vi "Set Editor Mode.vi"(8 "Error In":errorcluster, 10 "Mode in":T1, 11 "object in":refnum<class "WebView.JSONEditor.lvclass">) -> (0 "Error Out":errorcluster, 3 "object out":refnum<class "WebView.JSONEditor.lvclass">)   [LabVIEW 2020, in "WebView.JSONEditor.lvclass"]
uses:
  WebView.JSONEditor.lvclass
  <vilib>/JDP Science/JSONtext/LVClass Serializer/JSONtext LVClass Serializer.lvclass
  WebView_class/WebView.lvclass
  f8653de4-75b8-4eba-bbea-61abc822b106.vi
  WebView_class/Editor Mode--enum.ctl
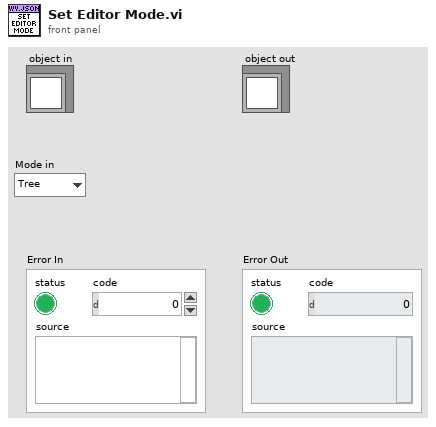
[diagram p1: front panel]
types:
  T1 = typedef "WebView.JSONEditor.lvclass/Editor Mode--enum.ctl" = enum16{"Tree", "View", "Form", "Code", "Text"}
  T2 = cluster{"type":enum16{"loadJSON", "setMode", "getJSON"}, "mode":string}
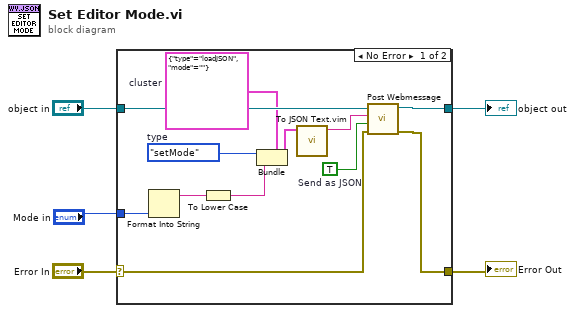
[diagram p0: block diagram]
diagram:
  n1 = case shown="No Error" "Error In" {
    selector: "Error In" -> [w8 w19]
    tunnel: [w7 w19] -> w4
    tunnel: [w14 w18] -> w2
    tunnel: "object in" -> [w15 w18]
    tunnel: "Mode in" -> [w17 _]
    frame No Error {
      w6 = T2 {"type"=enum."loadJSON", "mode"=""}  # cluster
      w9 = TRUE  # Send as JSON
      w13 = enum16{"loadJSON", "setMode", "getJSON"}."setMode"  # type
      n2 = Format Into String(w17) -> (resulting string=w16:string)  [unwired: 3 in, 1 out]
      n3 = To Lower Case(string=w16) -> (all lower case string=w12:string)
      n4 = Bundle(cluster=w6, "type"=w13, "mode"=w12) -> (w11:T2)
      n5 = call "To JSON Text.vim"("Anything"=w11) -> ("<JSON>"=w10:string)  [unwired: 9 in, 1 out]
      n6 = call "Post Webmessage.vi"("Error In"=w8, "Send as JSON"=w9, "Message"=w10, "WebView in"=w15) -> ("Error Out"=w7:errorcluster, "WebView out"=w14:refnum<class "WebView.JSONEditor.lvclass">)  [unwired: 6 in]
    }
    frame Error {
    }
  }
  "Error Out" <- w4
  "object out" <- w2
